vi "Test Get Account Data.vi"(8 "error in (no error)":errorcluster, 11 "Test Case In":refnum<class "Account Database Test.lvclass">) -> (0 "error out":errorcluster, 3 "Test Case Out":refnum<class "Account Database Test.lvclass">)   [LabVIEW 2020, in "Account Database Test.lvclass"]
uses:
  Account Database Test.lvclass
  Account Database Test.lvclass/Account Database Test.ctl
  Account Database/Account Database.lvclass
  Account Database/Account Data.ctl
  323c7dbb-e18d-4710-9182-97262e8b68d0.vi
  C:/Program Files (x86)/National Instruments/LabVIEW 2020/vi.lib/Astemes/LUnit/Test Case.lvclass
  C:/git/astemes-tdd-cld/source/Tests/Account Database Test/Account Database Test.lvclass
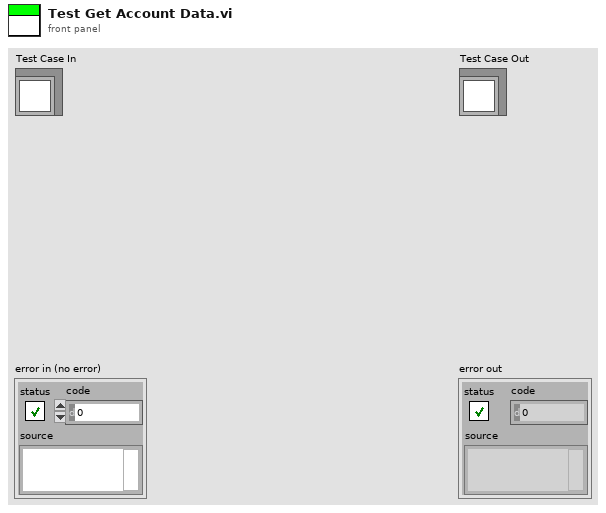
[diagram p1: front panel]
types:
  T1 = typedef "Account Database.lvclass/Account Data.ctl" = cluster{"Account Number":string, "First Name":string, "Last Name":string, "Account Balance":string}
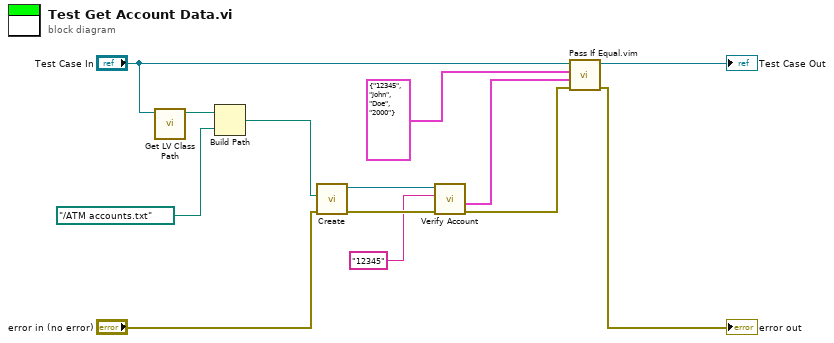
[diagram p0: block diagram]
diagram:
  n1 = call <vilib>:"Get LV Class Path.vi"("object"="Test Case In") -> ("class path"=w10:path)  [unwired: 9 in, 1 out]
  n2 = Build Path(base path=w10, name or relative path=path "../ATM accounts.txt") -> (appended path=w8:path)
  n3 = call "Create.vi"("error in (no error)"="error in (no error)", "Data File"=w8) -> ("error out"=w6:errorcluster, "Account Database out"=w4:refnum<class "Account Database.lvclass">)  [unwired: 8 in]
  n4 = call "Verify Account.vi"("error in (no error)"=w6, "Account Number"="12345", "Account Database in"=w4) -> ("error out"=w5:errorcluster, "Account Data"=w1:T1)  [unwired: 5 in, 2 out]
  n5 = call "Pass If Equal.vim"("error in (no error)"=w5, "Actual"=w1, "Expected"=T1 {"Account Number"="12345", "First Name"="John", "Last Name"="Doe", "Account Balance"="2000"} ("Account Data"), "LUnit Test Case In"="Test Case In") -> ("error out"=→"error out":errorcluster, "LUnit Test Case Out"=→"Test Case Out":refnum<class "Account Database Test.lvclass">)  [unwired: 6 in]
